vi "PositionCalculationLoop.vi"   [LabVIEW 2016]
uses:
  <vilib>/rvi/Emulation/niFpgaGetClockAttributes.vi
  <vilib>/rvi/Emulation/niFpgaSctlEmulationGetInTimedLoop.vi
  <vilib>/rvi/Emulation/niFpgaEmulationReportErrorSimple.vi
  <vilib>/rvi/Emulation/niFpgaEmulationIsFPGAContextNoSignature.vi
  <vilib>/rvi/errors/niFpgaSetErrorForExecOnDevCompSimple.vi
  <vilib>/rvi/eio/common/nirviEmuReportErrorAndStop.vi
  <vilib>/rvi/DataTransferAndStorage/Container/Common/niFpgaContainerGetUniqueNameForEmu.vi
  <vilib>/rvi/FIFO/Fifo_Resource/nirvififoEmulationSetSize.vi
  <vilib>/rvi/FIFO/Fifo_Resource/nirviFifoEmulationQueueMgr.vi
  <instcachedir>/0/nirviFifoEmulationQueueMgr_E5CAEC123FF24DC58D834DCA3CDAA9B5.lvgen/nirviFifoEmulationQueueMgr_E5CAEC123FF24DC58D834DCA3CDAA9B5_028.vi
  <vilib>/Utility/error.llb/Clear Errors.vi
  <vilib>/rvi/FIFO/Fifo_Resource/nirvififoEmulationCreateLock.vi
  <vilib>/rvi/Emulation/niFpgaProcessEmulError.vi
  <vilib>/rvi/FIFO/Fifo_Resource/nirvififoEmulationObtainLock.vi
  <vilib>/rvi/FIFO/Fifo_Resource/nirvififoEmulationReleaseLock.vi
  <vilib>/rvi/occurrence/nirviWaitOnOccurrenceBase.vi
  <vilib>/rvi/errors/nirviReportUnexpectedCaseInternalError.vi
  <vilib>/rvi/errors/nirviReportUnexpectedCaseInternalError (U32).vi
  <vilib>/rvi/Memory/Memory_Emulation/nirvimemoryFastEmulation.vi
  <vilib>/rvi/Memory/Memory_Emulation/nirvimemoryEmulation.vi
  <userlib>/_NI FLP Library/FPGA/outsideSCTL/FlpLib Multiply Shared Instance 0.vi
  <userlib>/_NI FLP Library/FPGA/outsideSCTL/FlpLib Add Shared Instance 0.vi
  <vilib>/rvi/FIFO/Fifo_Resource/nirvififoEmulationDetermineInputValidOut.vi
  <vilib>/rvi/Emulation/niFpgaCriticalErrorInLSC.vi
  <vilib>/rvi/DataTransferAndStorage/Container/XNode/niFpgaContainer.xnode
  <vilib>/rvi/FIFO/Fifo_Resource/nirvififoEmulationRead.vi
  <vilib>/rvi/FIFO/Fifo_Resource/nirvififoEmulationWrite.vi
types:
  T1 = cluster{"Timestamp":u64, "TxBytes":u64, "RxBytes":u64, "TxFrames":u64, "RxFrames":u64, "Sensor1Raw":i32, "Sensor2Raw":i32, "Sensor3Raw":i32, "Sensor4Raw":i32, "Sensor5Raw":i32, "Sensor6Raw":i32, "Sensor7Raw":i32, "Sensor8Raw":i32, "Sensor1Eng":sgl, "Sensor2Eng":sgl, "Sensor3Eng":sgl, "Sensor4Eng":sgl, "Sensor5Eng":sgl, "Sensor6Eng":sgl, "Sensor7Eng":sgl, "Sensor8Eng":sgl, "PositionX":sgl, "PositionY":sgl, "PositionZ":sgl, "RotationX":sgl, "RotationY":sgl, "RotationZ":sgl}
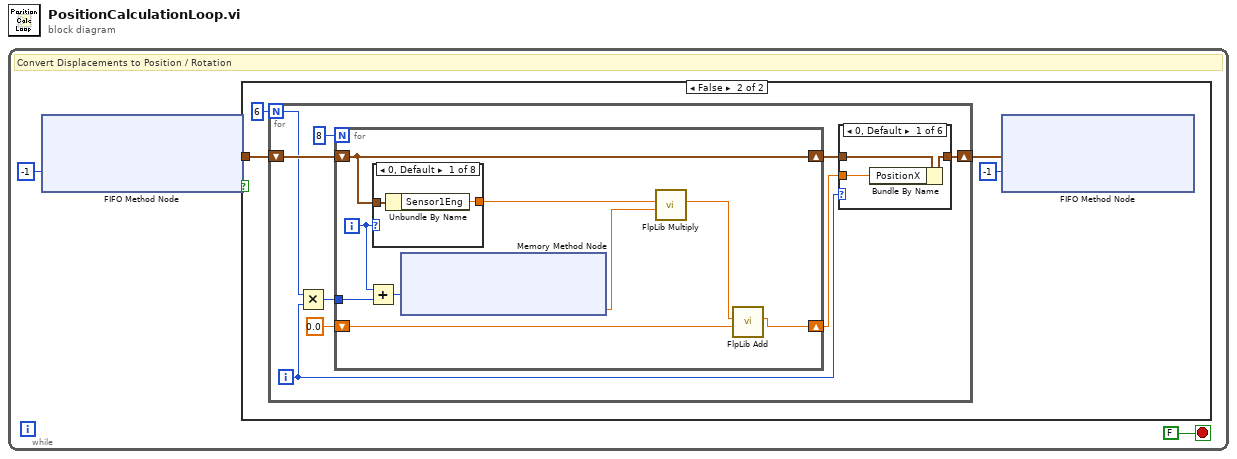
[diagram p0: block diagram]
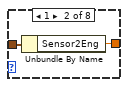
[diagram p3: hidden frame]
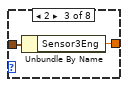
[diagram p4: hidden frame]
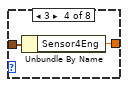
[diagram p5: hidden frame]
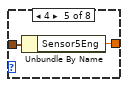
[diagram p6: hidden frame]
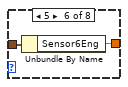
[diagram p7: hidden frame]
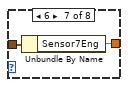
[diagram p8: hidden frame]
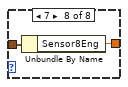
[diagram p9: hidden frame]
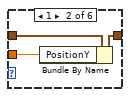
[diagram p10: hidden frame]
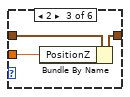
[diagram p11: hidden frame]
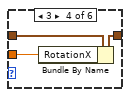
[diagram p12: hidden frame]
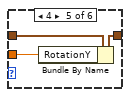
[diagram p13: hidden frame]
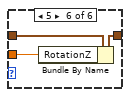
[diagram p14: hidden frame]
diagram:
  n1 = while {
    stop <- FALSE stop-if-true
    # "Convert Displacements to Position / Rotation"
    n2 = xnode ("FIFO Method Node")("Timeout"=-1) -> ("Element"=w2:T1, "Timed Out?"=w3:bool)  [unwired: 1 in, 1 out]
    n3 = case shown="False" w3 {
      tunnel: w2 -> [_ w6]
      frame True {
      }
      frame False {
        n4 = for {
          N: 6 -> [w13]
          shift-right: [w15] -> w5
          shift-left: w6 -> [w16]
          i -> [w14]
          n5 = Multiply(x=w13, y=w14) -> (x*y=w12:i32)
          n6 = for {
            N: 8 -> [_]
            shift-right: [w18] -> w10
            shift-left: w16 -> [w18]
            tunnel: w12 -> [w25]
            shift-right: [w19] -> w9
            shift-left: sgl 0.0 -> [w20]
            i -> [w26]
            n7 = Add(x=w26, y=w25) -> (x+y=w24:i32)
            n8 = case shown="0, Default" w26 {
              tunnel: w18 -> [w28 w30 w32 w34 w36 w38 w40 w42]
              tunnel: [w27 w29 w31 w33 w35 w37 w39 w41] -> w22
              frame 0, Default {
                n9 = Unbundle By Name(w28) -> ("Sensor1Eng"=w27:sgl)
              }
              frame 1 {
                n10 = Unbundle By Name(w30) -> ("Sensor2Eng"=w29:sgl)
              }
              frame 2 {
                n11 = Unbundle By Name(w32) -> ("Sensor3Eng"=w31:sgl)
              }
              frame 3 {
                n12 = Unbundle By Name(w34) -> ("Sensor4Eng"=w33:sgl)
              }
              frame 4 {
                n13 = Unbundle By Name(w36) -> ("Sensor5Eng"=w35:sgl)
              }
              frame 5 {
                n14 = Unbundle By Name(w38) -> ("Sensor6Eng"=w37:sgl)
              }
              frame 6 {
                n15 = Unbundle By Name(w40) -> ("Sensor7Eng"=w39:sgl)
              }
              frame 7 {
                n16 = Unbundle By Name(w42) -> ("Sensor8Eng"=w41:sgl)
              }
            }
            n17 = xnode ("Memory Method Node")("Address"=w24) -> ("Data"=w23:sgl)  [unwired: 1 in, 1 out]
            n18 = call-poly <userlib>:"FlpLib Multiply.vi"("y"=w23, "x"=w22) -> ("x*y"=w21:sgl)  [unwired: 5 in]
            n19 = call-poly <userlib>:"FlpLib Add.vi"("y"=w20, "x"=w21) -> ("x+y"=w19:sgl)  [unwired: 5 in]
          }
          n20 = case shown="0, Default" w14 {
            tunnel: w10 -> [w45 w48 w51 w54 w57 w60]
            tunnel: [w44 w47 w50 w53 w56 w59] -> w15
            tunnel: w9 -> [w43 w46 w49 w52 w55 w58]
            frame 0, Default {
              n21 = Bundle By Name(cluster=w45, "PositionX"=w43) -> (w44:T1)
            }
            frame 1 {
              n22 = Bundle By Name(cluster=w48, "PositionY"=w46) -> (w47:T1)
            }
            frame 2 {
              n23 = Bundle By Name(cluster=w51, "PositionZ"=w49) -> (w50:T1)
            }
            frame 3 {
              n24 = Bundle By Name(cluster=w54, "RotationX"=w52) -> (w53:T1)
            }
            frame 4 {
              n25 = Bundle By Name(cluster=w57, "RotationY"=w55) -> (w56:T1)
            }
            frame 5 {
              n26 = Bundle By Name(cluster=w60, "RotationZ"=w58) -> (w59:T1)
            }
          }
        }
        n27 = xnode ("FIFO Method Node")("Element"=w5, "Timeout"=-1) -> ()  [unwired: 1 in, 2 out]
      }
    }
  }
